vi "Control Panel.vi"(8 "error in (no error)":errorcluster, 11 "Fake Power Meter in":refnum<class "Power Meter.lvclass">) -> (0 "error out":errorcluster, 3 "Fake Power Meter out":refnum<class "Power Meter.lvclass">)   [LabVIEW 2009, in "Power Meter.lvclass"]
doc: "(Dynamic) A user-level application that simulates the physical front panel of the Instrument. Provide the user with buttons to manually control features of the instrument, and provide indicators of its current state."
uses:
  Power Meter.lvclass
  Utility Classes/Readable/Readable.lvclass
  Power Meter.lvclass/Power Meter.ctl
panel:
  in  "Averaging Time":dbl=0.5
  in  "Averaging":bool
  out "Units":u16(ring) items=["W"=1, "dB"=2, "dBm"=3, "REL"=4]
  out "AVG":u16(ring) items=["Slow"=1, "Medium"=2, "Fast"=3]
  out "Run/Stop":u16(ring) items=["Stop", "Run"]
  out "ATTN":u16(ring) items=["Off", "On"]
  out "Local Lockout":u16(ring) items=["Off", "On"]
  out "Zero":u16(ring) items=["Off", "On"]
  out "Beeper":u16(ring) items=["Off", "On"]
  out "Backlight":u16(ring) items=["Off", "Low", "High"]
  out "Range":u16(ring) items=["Auto", "Lowest", "2", "3", "4", "5", "6", "7", "Highest"]
  in  "Run/Stop set":u32(ring)=1 items=["Stop", "Run"]
  in  "ATTN set":u32(ring) items=["Off", "On"]
  in  "BKLT set":u32(ring)=1 items=["Off", "Low", "High"]
  in  "Range set":u32(ring) items=["Auto", "Lowest", "2", "3", "4", "5", "6", "7", "Highest"]
  in  "Beeper set":u32(ring) items=["Off", "On"]
  in  "AVG set":u32(ring)=2 items=["Slow"=1, "Medium"=2, "Fast"=3]
  in  "Units set":u32(ring)=1 items=["W"=1, "dB"=2, "mdB"=3, "REL"=4]
  in  "Zero set":u32(ring) items=["Off", "On"]
  in  "Local set":u32(ring) items=["Off", "On"]
  in  "Read Current Value":bool
  out "Value":dbl
  in  "Set":bool
  in  "Read to Control":bool
  in  "Read":bool
  in  "Wavelength Set":dbl[unit]
  out "Wavelength":dbl[unit]
  in  "Copy actual to set":bool
  in  "Populate fields with member data":bool
  in  "stop":bool
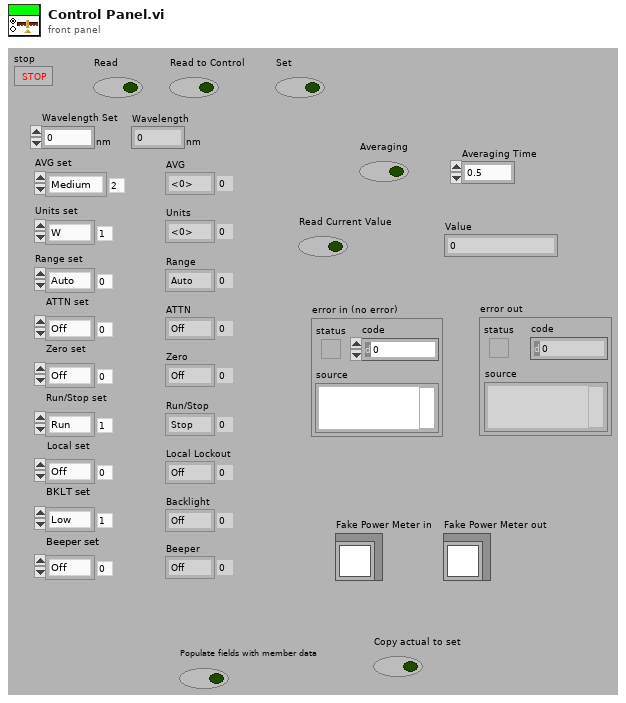
[diagram p1: front panel]
types:
  T1 = typedef "Readable.lvclass/X array.ctl" = T2[]
  T2 = typedef "Readable.lvclass/X.ctl" = dbl
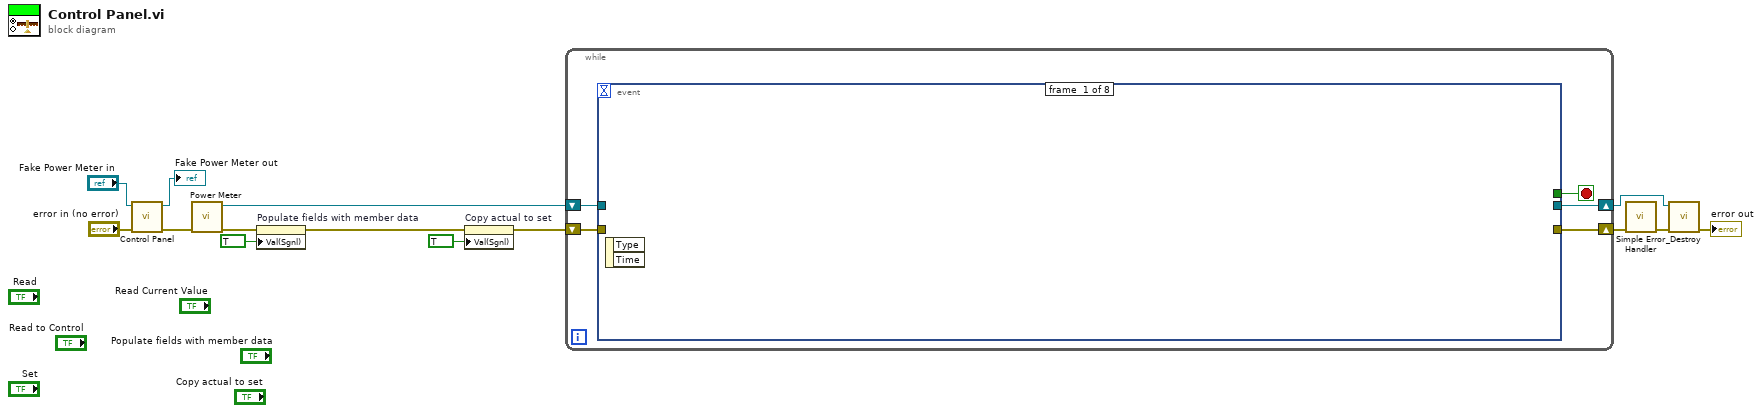
[diagram p0: block diagram]
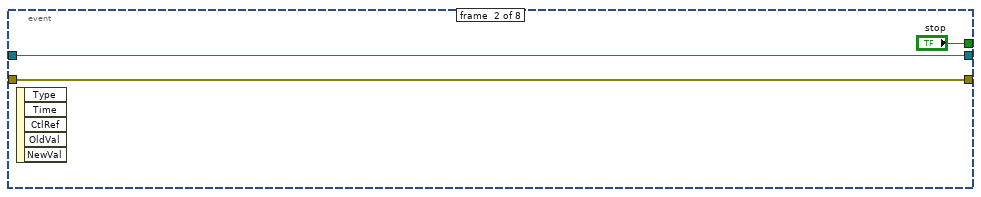
[diagram p2: hidden frame]
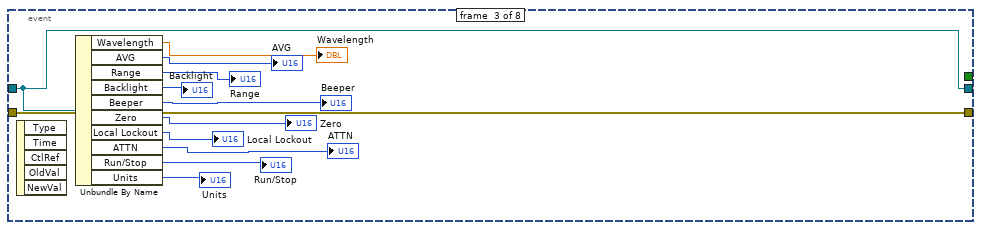
[diagram p3: hidden frame]
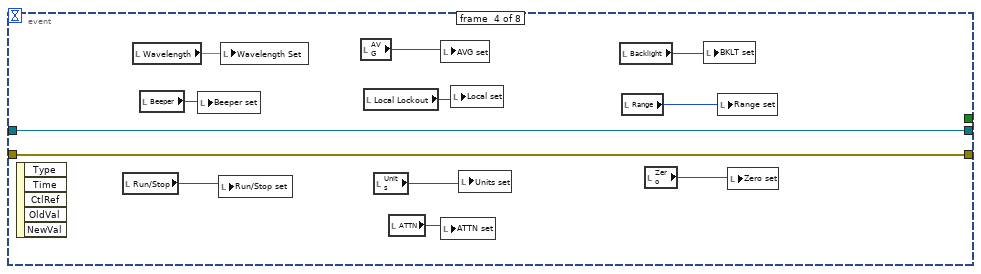
[diagram p4: hidden frame]
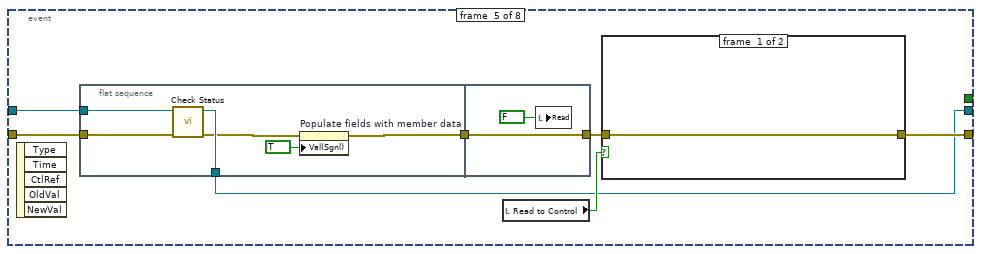
[diagram p5: hidden frame]
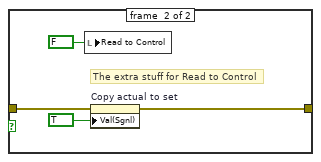
[diagram p6: hidden frame]
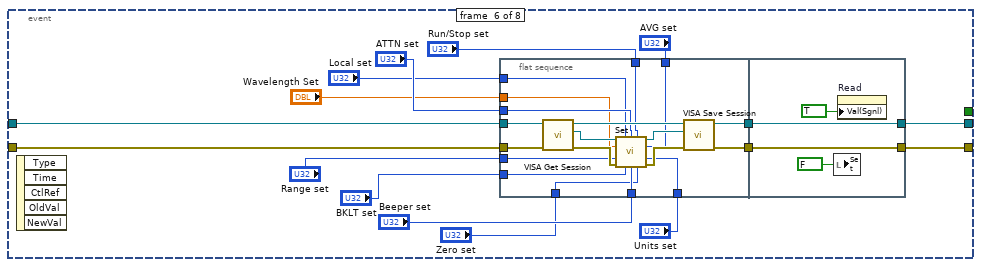
[diagram p7: hidden frame]
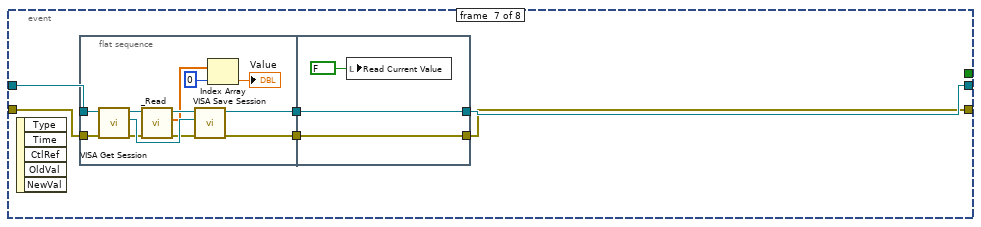
[diagram p8: hidden frame]
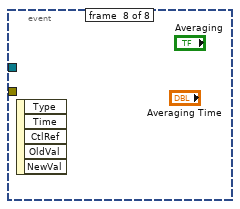
[diagram p9: hidden frame]
diagram:
  n1 = call-parent "Control Panel.vi"("error in (no error)"="error in (no error)", "Instrument in"="Fake Power Meter in") -> ("error out"=w12:errorcluster, "Instrument out"=→"Fake Power Meter out":refnum<class "Power Meter.lvclass">)  [unwired: 8 in]
  n2 = call "Power Meter.vi"("error in (no error)"=w12) -> ("error out"=w6:errorcluster, "Power Meter out"=w11:refnum<class "Power Meter.lvclass">)  [unwired: 9 in]
  n3 = property on="Populate fields with member data" class="Bool (strict)"(error in=w6, "Val(Sgnl)"=TRUE ("Value (Signaling)")) -> (error out=w7:errorcluster)  [unwired: 1 in, 1 out]
  n4 = property on="Copy actual to set" class="Bool (strict)"(error in=w7, "Val(Sgnl)"=TRUE ("Value (Signaling)")) -> (error out=w5:errorcluster)  [unwired: 1 in, 1 out]
  n5 = while {
    shift-right: [w16] -> w4
    shift-left: w11 -> [w18]
    shift-right: [w15] -> w3
    shift-left: w5 -> [w17]
    stop <- w19 stop-if-true
    n6 = event shown="[7] \"Averaging\", \"Averaging Time\": Value Change" {
      selector: _ -> [_ _ _ _ _ _ _ _]
      dyn-events: _ -> [_ _ _ _ _ _ _ _]
      timeout: _ -> [_ _ _ _ _ _ _ _]
      tunnel: [_ "stop" _ _ _ _ _ _] -> w19
      tunnel: [_ w21 w33 w45 w47 w78 w107 _] -> w16
      tunnel: w18 -> [_ w21 w33 w45 w53 w81 w111 _]
      tunnel: [_ w20 w32 w44 w48 w77 w106 _] -> w15
      tunnel: w17 -> [_ w20 w32 w44 w52 w79 w109 _]
      event #0 {
        n7 = event-data() -> ()  [unwired: 1 in, 2 out]
      }
      event #1 {
        n8 = event-data() -> ()  [unwired: 1 in, 5 out]
      }
      event #2 {
        n9 = event-data() -> ()  [unwired: 1 in, 5 out]
        n10 = Unbundle By Name(w33) -> ("Wavelength"=→"Wavelength":dbl[unit], "AVG"=→"AVG":u16, "Range"=→"Range":u16, "Backlight"=→"Backlight":u16, "Beeper"=→"Beeper":u16, "Zero"=→"Zero":u16, "Local Lockout"=→"Local Lockout":u16, "ATTN"=→"ATTN":u16, "Run/Stop"=→"Run/Stop":u16, "Units"=→"Units":u16)
      }
      event #3 {
        n11 = event-data() -> ()  [unwired: 1 in, 5 out]
        n12 = local read "Run/Stop"() -> (w38:u16)
        n13 = local read "Wavelength"() -> (w46:dbl[unit])
        n14 = local read "Beeper"() -> (w41:u16)
        n15 = local write "Beeper set"(w41) -> ()
        n16 = local write "Run/Stop set"(w38) -> ()
        n17 = local write "Wavelength Set"(w46) -> ()
        n18 = local read "AVG"() -> (w43:u16)
        n19 = local read "Local Lockout"() -> (w40:u16)
        n20 = local read "Units"() -> (w37:u16)
        n21 = local read "ATTN"() -> (w36:u16)
        n22 = local write "AVG set"(w43) -> ()
        n23 = local write "ATTN set"(w36) -> ()
        n24 = local write "Local set"(w40) -> ()
        n25 = local write "Units set"(w37) -> ()
        n26 = local read "Backlight"() -> (w42:u16)
        n27 = local read "Range"() -> (w39:u16)
        n28 = local read "Zero"() -> (w35:u16)
        n29 = local write "BKLT set"(w42) -> ()
        n30 = local write "Range set"(w39) -> ()
        n31 = local write "Zero set"(w35) -> ()
      }
      event #4 {
        n32 = event-data() -> ()  [unwired: 1 in, 5 out]
        n33 = flat-sequence {
          tunnel: w53 -> [w64]
          tunnel: w52 -> [w63]
          tunnel: [w60] -> w49
          tunnel: [w62] -> w47
          tunnel: [w65] -> w50
          tunnel: w49 -> [w65]
          frame #0 {
            n34 = call-dynamic "Check Status.vi"("error in (no error)"=w63, "Power Meter in"=w64) -> ("error out"=w61:errorcluster, "Power Meter out"=w62:refnum<class "Power Meter.lvclass">)  [unwired: 6 in, 2 out]
            n35 = property on="Populate fields with member data" class="Bool (strict)"(error in=w61, "Val(Sgnl)"=TRUE ("Value (Signaling)")) -> (error out=w60:errorcluster)  [unwired: 1 in, 1 out]
          }
          frame #1 {
            n36 = local write "Read"(FALSE ("Read")) -> ()
          }
        }
        n37 = local read "Read to Control"() -> (w51:bool)
        n38 = case shown="True" w51 {
          tunnel: w50 -> [w54 w56]
          tunnel: [w54 w55] -> w48
          frame #0 {
          }
          frame #1 {
            # "The extra stuff for Read to Control"
            n39 = local write "Read to Control"(FALSE ("Read")) -> ()
            n40 = property on="Copy actual to set" class="Bool (strict)"(error in=w56, "Val(Sgnl)"=TRUE ("Value (Signaling)")) -> (error out=w55:errorcluster)  [unwired: 1 in, 1 out]
          }
        }
      }
      event #5 {
        n41 = event-data() -> ()  [unwired: 1 in, 5 out]
        n42 = flat-sequence {
          tunnel: [w99] -> w82
          tunnel: w81 -> [w100]
          tunnel: [w97] -> w80
          tunnel: w79 -> [w98]
          tunnel: "AVG set" -> [w92]
          tunnel: "Units set" -> [w91]
          tunnel: "Run/Stop set" -> [w90]
          tunnel: "ATTN set" -> [w89]
          tunnel: "Local set" -> [w88]
          tunnel: "Wavelength Set" -> [w87]
          tunnel: "Range set" -> [w86]
          tunnel: "BKLT set" -> [w85]
          tunnel: "Beeper set" -> [w84]
          tunnel: "Zero set" -> [w83]
          tunnel: [w103] -> w78
          tunnel: w82 -> [w103]
          tunnel: [w102] -> w77
          tunnel: w80 -> [w102]
          frame #0 {
            n43 = call-dynamic "VISA Get Session.vi"("error in (no error)"=w98, "Instrument.lvclass in"=w100) -> ("error out"=w93:errorcluster, "VISA Resource Name"=w96:refnum<visa-resource-name>, "Instrument.lvclass out"=w101:refnum<class "Power Meter.lvclass">)  [unwired: 7 out]
            n44 = call "Set.vi"("VISA resource name"=w96, "Local Lockout (0:1)"=w88, "ATTN (0:1)"=w89, "Run/Stop (1:0)"=w90, "Wavelength (nnnn)"=w87, "AVG (1:3)"=w92, "Range (0-Auto,1:8)"=w86, "Units (1:4)"=w91, "error in (no error)"=w93, "Backlight (0:2)"=w85, "Beeper (0:1)"=w84, "Zero (0:1)"=w83) -> ("VISA resource name out"=w95:refnum<visa-resource-name>, "error out"=w94:errorcluster)  [unwired: 2 in]
            n45 = call-dynamic "VISA Save Session.vi"("error in (no error)"=w94, "VISA Resource Name"=w95, "Instrument.lvclass in"=w101) -> ("error out"=w97:errorcluster, "Instrument.lvclass out"=w99:refnum<class "Power Meter.lvclass">)  [unwired: 7 out]
          }
          frame #1 {
            n46 = local write "Set"(FALSE ("Set")) -> ()
            n47 = property on="Read" class="Bool (strict)"("Val(Sgnl)"=TRUE ("Value (Signaling)")) -> ()  [unwired: 2 in, 2 out]
          }
        }
      }
      event #6 {
        n48 = event-data() -> ()  [unwired: 1 in, 5 out]
        n49 = flat-sequence {
          tunnel: w111 -> [w123]
          tunnel: [w122] -> w110
          tunnel: w109 -> [w121]
          tunnel: [w120] -> w108
          tunnel: [w125] -> w107
          tunnel: w110 -> [w125]
          tunnel: [w124] -> w106
          tunnel: w108 -> [w124]
          frame #0 {
            n50 = call-dynamic "VISA Get Session.vi"("error in (no error)"=w121, "Instrument.lvclass in"=w123) -> ("error out"=w116:errorcluster, "VISA Resource Name"=w119:refnum<visa-resource-name>, "Instrument.lvclass out"=w118:refnum<class "Power Meter.lvclass">)  [unwired: 7 out]
            n51 = call-dynamic "_Read.vi"("error in (no error)"=w116, "Power Meter in"=w118) -> ("error out"=w115:errorcluster, "X array"=w114:T1, "Power Meter out"=w117:refnum<class "Power Meter.lvclass">)  [unwired: 7 in]
            n52 = call-dynamic "VISA Save Session.vi"("error in (no error)"=w115, "VISA Resource Name"=w119, "Instrument.lvclass in"=w117) -> ("error out"=w120:errorcluster, "Instrument.lvclass out"=w122:refnum<class "Power Meter.lvclass">)  [unwired: 7 out]
            n53 = Index Array(array=w114, index=0) -> (element=→"Value":T2)
          }
          frame #1 {
            n54 = local write "Read Current Value"(FALSE ("Read Current Value")) -> ()
          }
        }
      }
      event #7 {
        n55 = event-data() -> ()  [unwired: 1 in, 5 out]
      }
    }
  }
  n56 = call <vilib>:"Simple Error Handler.vi"("error in (no error)"=w3) -> ("error out"=w2:errorcluster)  [unwired: 1 in, 7 out]
  n57 = call-dynamic "_Destroy.vi"("error in (no error)"=w2, "Instrument in"=w4) -> ("error out"=→"error out":errorcluster)  [unwired: 9 out]
